vi "locate all system variables.vi"(8 "error in":errorcluster) -> (0 "error out":errorcluster, 3 "system variables":T1[](array[typedef]))   [LabVIEW 2013, in "Scan Engine runtime.lvclass"]
uses:
  Scan Engine runtime.lvclass
  Custom Ctrls/system variable.ctl
  <vilib>/NI/Tag Bus/tag/Data Type.ctl
  <vilib>/Utility/VariantDataType/VariantType.lvlib
  <resource>/objmgr/ni.var.rc
  <vilib>/NI/Tag Bus/tag/tag descriptor.lvclass
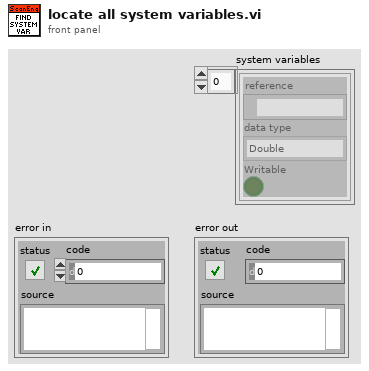
[diagram p1: front panel]
types:
  T1 = typedef "Scan Engine runtime.lvclass/system variable.ctl" = cluster{"reference":refnum<k21>, "data type":T2, "Writable":bool}
  T2 = typedef "tag bus.lvlib/tag descriptor.lvclass/Data Type.ctl" = enum16{"Double", "Single", "I64", "I32", "I16", "I8", "U64", "U32", "U16", "U8", "Boolean", "String", "Array of Double", "Array of Single", "Array of I64", "Array of I32", "Array of I16", "Array of I8", "Array of U64", "Array of U32", "Array of U16", "Array of U8", "Array of Boolean", "Array of String"}
  T3 = typedef "VariantType.lvlib/Type.ctl" = enum8{"Invalid Type", "Void", "I8", "I16", "I32", "I64", "U8", "U16", "U32", "U64", "Single Float", "Double Float", "Extended Float", "Single Complex", "Double Complex", "Extended Complex", "Enum U8", "Enum U16", "Enum U32", "Enum U64", "Single Float With Unit", "Double Float With Unit", "Extended Float With Unit", "Single Complex with Unit", "Double Complex with Unit", "Extended Complex with Unit", "Boolean", "String", "Path", "Picture", "Tag", "Array", "Cluster", "Variant", "LV Variant", "Waveform", "Timestamp", "Digital Waveform", "Digital Data", "ExpressData", "Refnum", "External Data", "VI", "Poly VI", "LabVIEW Class Instance", "Fixed Point"}
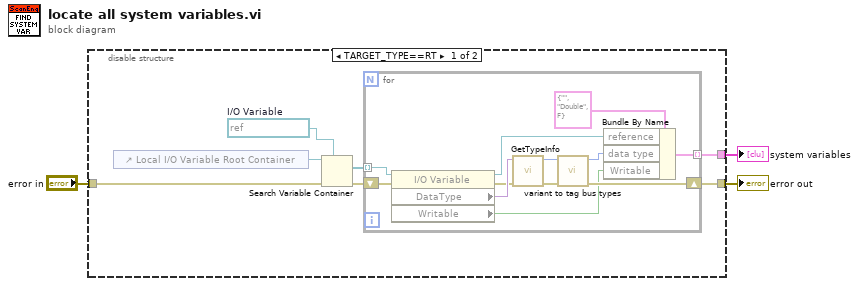
[diagram p0: block diagram]
diagram:
  n1 = disable-structure shown="TARGET_TYPE==RT" {
    disable-tunnel: [w10 w22] -> w3
    disable-tunnel: "error in" -> [w8 w22]
    disable-tunnel: [w4 _] -> w1
    frame condition #0 {
      w6 = refnum<k21> refnum  # I/O Variable
      n2 = control-ref of="Local I/O Variable Root Container"() -> (w7:refnum<k21>)
      n3 = Search Variable Container(7:w6, 8:w8, 11:w7) -> (0:w9:errorcluster, 2:w5:refnum<k21>[])  [unwired: 3 in, 1 out]
      n4 = for {
        shift-right: [w19] -> w10
        shift-left: w9 -> [w20]
        tunnel: w5 -> [w21] mode=indexing
        tunnel: [w18] -> w4 mode=indexing
        n5 = property class="I/O Variable"(reference=w21, error in=w20) -> (reference out=w15:refnum<k21>, error out=w16:errorcluster, "DataType"=w17:variant, "Writable"=w14:bool)
        n6 = call <vilib>:"GetTypeInfo.vi"("error in (no error)"=w16, "Variant"=w17) -> ("error out"=w19:errorcluster, "Type Enum"=w12:T3)  [unwired: 5 in, 3 out]
        n7 = call "variant to tag bus types.vi"("Type Enum"=w12) -> ("data type"=w11:T2)  [unwired: 10 in]
        n8 = Bundle By Name(cluster=T1 {"reference"="", "data type"=enum."Double", "Writable"=FALSE} ("raw variable data"), "reference"=w15, "data type"=w11, "Writable"=w14) -> (w18:T1)
      }
    }
    frame condition #1 (active) {
    }
  }
  "error out" <- w3
  "system variables" <- w1
